vi "Inspect Elements in Memory.vi"(8 "error in (no error)":errorcluster, 10 "Size Info":T1, 11 "CIPC Reference":u64) -> (0 "error out":errorcluster, 1 "Oldest Index":u32, 2 "Newest Index":u32, 3 "Next Read Index":u32, 5 "Next Not Available":bool)   [LabVIEW 2021, in "CIF_NI_CIPC.lvlib"]
doc: "Check the number of elements available in the buffer.\n\nOutputs:\n- el_index_next_read: element index from which the next element will be read\n- el_index_newest: most recent element index available in memory\n- el_index_oldest: oldest element index available in memory\n- next_not_available: boolean indicating if the next element to read is available in memory"
uses:
  CIF_NI_CIPC.lvlib
  TypeDefs/Info Size.ctl
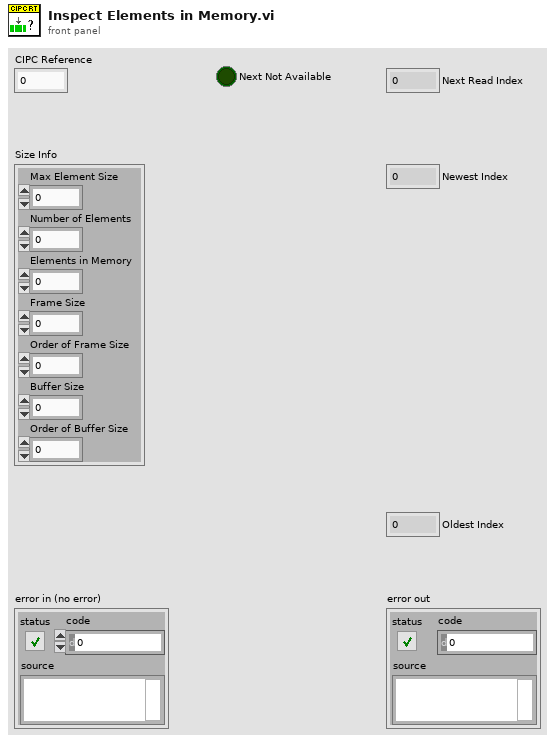
[diagram p1: front panel]
types:
  T1 = typedef "CIF_NI_CIPC.lvlib/Info Size.ctl" = cluster{"Max Element Size":u32, "Number of Elements":u32, "Elements in Memory":u32, "Frame Size":u32, "Order of Frame Size":u32, "Buffer Size":u32, "Order of Buffer Size":u32}
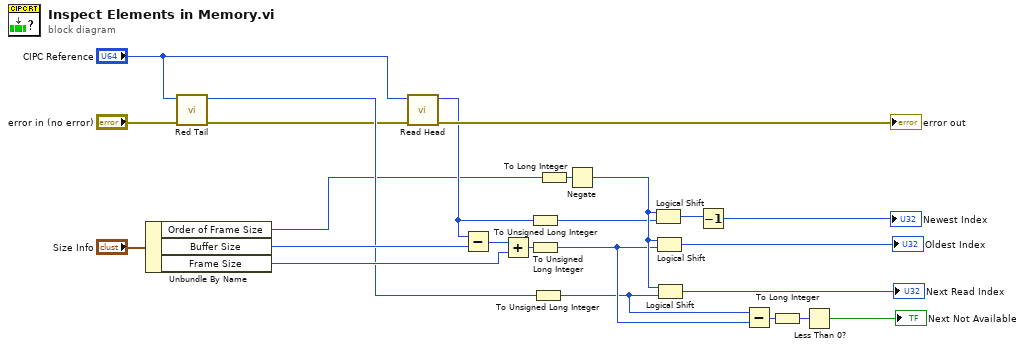
[diagram p0: block diagram]
diagram:
  n1 = Unbundle By Name("Size Info") -> ("Order of Frame Size"=w1:u32, "Buffer Size"=w22:u32, "Frame Size"=w8:u32)
  n2 = call "Red Tail.vi"("error in (no error)"="error in (no error)", "CIPC Reference"="CIPC Reference") -> ("error out"=w5:errorcluster, "Tail"=w6:u32)  [unwired: 8 in]
  n3 = call "Read Head.vi"("error in (no error)"=w5, "CIPC Reference"="CIPC Reference") -> ("error out"=→"error out":errorcluster, "Head"=w18:u32)  [unwired: 8 in]
  n4 = Subtract(x=w18, y=w22) -> (x-y=w9:u32)
  n5 = Add(x=w9, y=w8) -> (x+y=w7:u32)
  n6 = To Unsigned Long Integer(number=w18) -> (unsigned 32bit integer=w17:u32)
  n7 = To Unsigned Long Integer(number=w7) -> (unsigned 32bit integer=w11:u32)
  n8 = To Unsigned Long Integer(number=w6) -> (unsigned 32bit integer=w10:u32)
  n9 = To Long Integer(number=w1) -> (32bit integer=w24:i32)
  n10 = Negate(x=w24) -> (-x=w21:i32)
  n11 = Logical Shift(y=w21, x=w17) -> (x << y=w20:u32)
  n12 = Logical Shift(y=w21, x=w11) -> (x << y=→"Oldest Index":u32)
  n13 = Logical Shift(y=w21, x=w10) -> (x << y=→"Next Read Index":u32)
  n14 = Decrement(x=w20) -> (x-1=→"Newest Index":u32)
  n15 = Subtract(x=w10, y=w11) -> (x-y=w14:u32)
  n16 = To Long Integer(number=w14) -> (32bit integer=w13:i32)
  n17 = Less Than 0?(x=w13) -> (x < 0?=→"Next Not Available":bool)
